vi "Main.vi"() -> ()   [LabVIEW 2020]
uses:
  <vilib>/DAQmx/read.llb/DAQmx Read (Analog DBL 1Chan 1Samp).vi
  <vilib>/DAQmx/create/channels.llb/DAQmx Create Channel (AI-Temperature-Thermocouple).vi
  <vilib>/DAQmx/configure/timing.llb/DAQmx Timing (Sample Clock).vi
  <vilib>/DAQmx/miscellaneous.llb/DAQmx Fill In Error Info.vi
panel:
  out "Weather Data":T1
  out "Waveform Chart":dbl(graph)
  in  "Stop":bool
  in  "Lower Limit":dbl=20.0
  in  "Upper Limit":dbl=30.0
  in  "Thermocouple Channel":tag="PCI-6221/ai0"
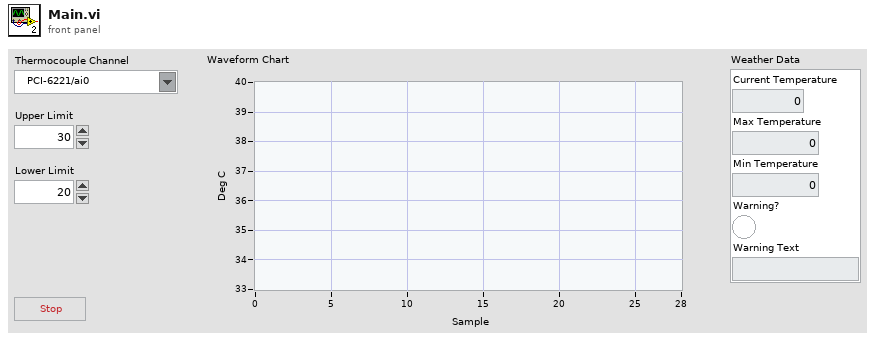
[diagram p1: front panel]
types:
  T1 = cluster{"Current Temperature":dbl, "Max Temperature":dbl, "Min Temperature":dbl, "Warning?":bool, "Warning Text":string}
  T2 = enum16{"open", "replace", "create", "open or create", "replace or create", "replace or create with confirmation"}
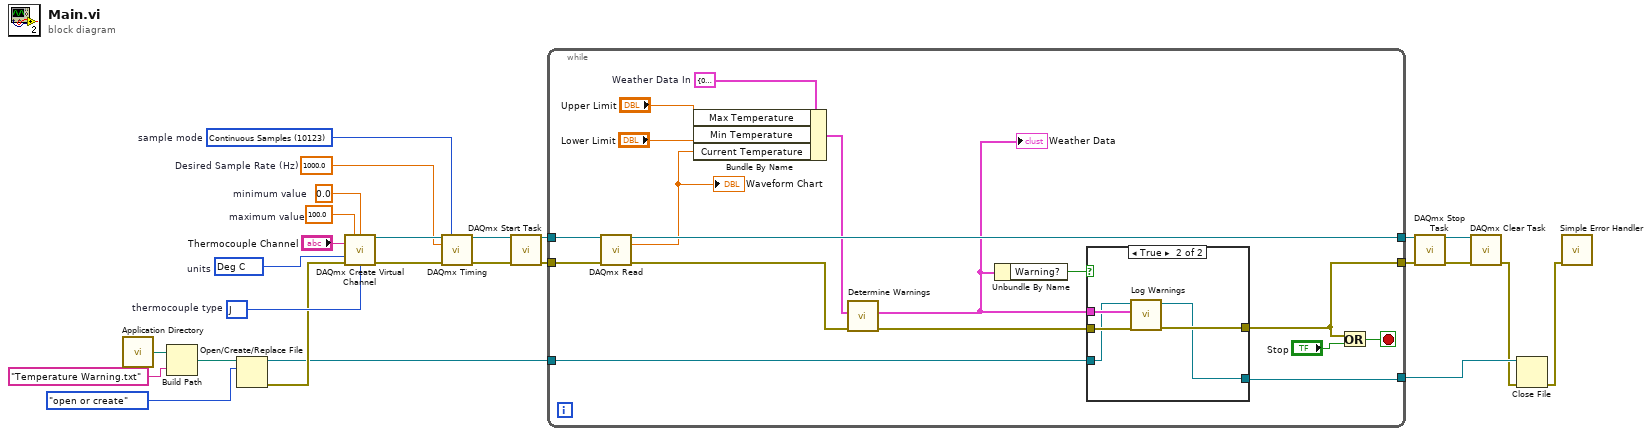
[diagram p0: block diagram]
diagram:
  w13 = 1000.0  # Desired Sample Rate (Hz)
  w14 = 10123 items=["Finite Samples"=10178, "Continuous Samples"=10123, "Hardware Timed Single Point"=12522]  # sample mode
  w22 = 10143 items=["Deg C"=10143, "Deg F"=10144, "Kelvins"=10325, "Deg R"=10145, "From Custom Scale"=10065]  # units
  w23 = 10072 items=["J"=10072, "K"=10073, "N"=10077, "R"=10082, "S"=10085, "T"=10086, "B"=10047, "E"=10055]  # thermocouple type
  w24 = 100.0  # maximum value
  w25 = 0.0  # minimum value
  n1 = call <vilib>:"Application Directory.vi"() -> ("Application Directory"=w21:path)
  n2 = Build Path(base path=w21, name or relative path="Temperature Warning.txt") -> (appended path=w19:path)
  n3 = Open/Create/Replace File(file path (use dialog)=w19, operation (0:open)=T2."open or create") -> (refnum out=w8:refnum<file>, error out=w17:errorcluster)  [unwired: 4 in, 1 out]
  n4 = call-poly <vilib>:"DAQmx Create Virtual Channel.vi"("maximum value"=w24, "minimum value"=w25, "physical channels"="Thermocouple Channel", "units"=w22, "error in"=w17, "thermocouple type"=w23) -> ("task out"=w16:refnum<k21>, "error out"=w15:errorcluster)  [unwired: 8 in]
  n5 = call-poly <vilib>:"DAQmx Timing.vi"("task/channels in"=w16, "sample mode"=w14, "rate"=w13, "error in"=w15) -> ("task out"=w12:refnum<k21>, "error out"=w11:errorcluster)  [unwired: 10 in]
  n6 = call <vilib>:"DAQmx Start Task.vi"("task/channels in"=w12, "error in"=w11) -> ("task out"=w10:refnum<k21>, "error out"=w9:errorcluster)  [unwired: 12 in]
  n7 = while {
    tunnel: w10 -> [w43]
    tunnel: w9 -> [w42]
    tunnel: [w41] -> w7
    tunnel: w8 -> [w34]
    tunnel: [w30] -> w3
    tunnel: [w27] -> w6
    stop <- w28 stop-if-true
    w40 = T1 {"Current Temperature"=0.0, "Max Temperature"=0.0, "Min Temperature"=0.0, "Warning?"=FALSE, "Warning Text"=""}  # Weather Data In
    n8 = call-poly <vilib>:"DAQmx Read.vi"("task/channels in"=w43, "error in"=w42) -> ("task out"=w41:refnum<k21>, "data"=w37:dbl, "error out"=w35:errorcluster)  [unwired: 11 in]
    "Waveform Chart" <- w37
    n9 = Bundle By Name(cluster=w40, "Max Temperature"="Upper Limit", "Min Temperature"="Lower Limit", "Current Temperature"=w37) -> (w36:T1)
    n10 = call "Determine Warnings.vi"("Error In"=w35, "Weather Data In"=w36) -> ("Error Out"=w31:errorcluster, "Weather Data Out"=w32:T1)  [unwired: 6 in]
    "Weather Data" <- w32
    n11 = Unbundle By Name(w32) -> ("Warning?"=w33:bool)
    n12 = case shown="True" w33 {
      tunnel: w34 -> [w44 w47]
      tunnel: w32 -> [_ w50]
      tunnel: w31 -> [w45 w49]
      tunnel: [w45 w48] -> w27
      tunnel: [w44 w46] -> w30
      frame False {
      }
      frame True {
        n13 = call "Log Warnings.vi"("Error In"=w49, "Weather Data"=w50, "file ref in"=w47) -> ("Error Out"=w48:errorcluster, "file ref out"=w46:refnum<file>)  [unwired: 7 in]
      }
    }
    n14 = Or(x=w27, y="Stop") -> (x .or. y?=w28:bool)
  }
  n15 = call <vilib>:"DAQmx Stop Task.vi"("task/channels in"=w7, "error in"=w6) -> ("task out"=w5:refnum<k21>, "error out"=w4:errorcluster)  [unwired: 12 in]
  n16 = call <vilib>:"DAQmx Clear Task.vi"("task in"=w5, "error in"=w4) -> ("error out"=w2:errorcluster)  [unwired: 13 in]
  n17 = Close File(refnum=w3, error in=w2) -> (error out=w1:errorcluster)  [unwired: 1 out]
  n18 = call <vilib>:"Simple Error Handler.vi"("error in (no error)"=w1) -> ()  [unwired: 4 in, 5 out]
